vi "PTC_FinalDemo.vi"() -> ()   [LabVIEW 2016]
uses:
  VIs/uPythonX/uPythonX.xctl
panel:
  in  "VISA resource name":refnum<visa-resource-name>
  in  "Thingworx":T1(xcontrol)={"VISA Refnum in"="pyboard - ASRL96::INSTR", "Python Code"="import machine, utime\nimport InternetClass, GroveClasses\n\nmachine.Pin('EN_3V3').on()\n       \nconnection = InternetClass.wifi()\n\n'''\ntemp = GroveClasses.GroveTemp('W24')\n\nwhile True:\n     temperature = temp.value()\n     print ('%4.2f' % (temperature))\n     if not connection.TW_Put('Spike', 'temperature1','NUMBER',str(temperature)):\n          utime.sleep(2)\n     else:\n          utime.sleep_ms(200)\n'''\nsound = GroveClasses.GroveSPL('W24')\n\nwhile True:\n     SPL = 0\n     size = 100\n     for i in range(size):\n          SPL += sound.value()/40.96\n     SPL /= size\n     print ('%4.2f' % (SPL))\n     if not connection.TW_Put('Spike', 'temperature2','NUMBER',str(SPL)):\n          utime.sleep(2)\n     else:\n          utime.sleep_ms(200)\n     \n"}
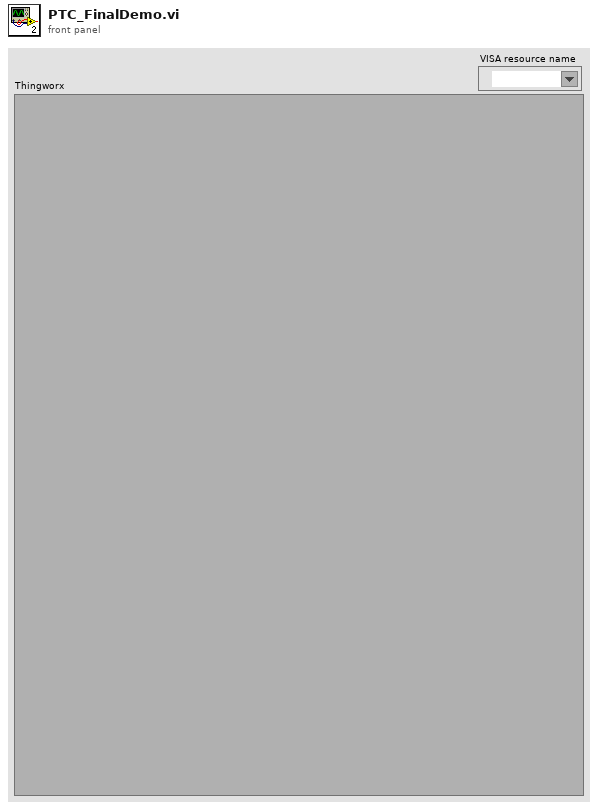
[diagram p1: front panel]
types:
  T1 = cluster{"VISA Refnum in":refnum<visa-resource-name>, "Python Code":string}
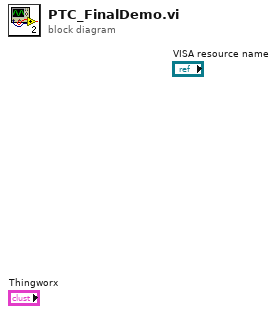
[diagram p0: block diagram]
diagram:
